vi "Calc Batch Profile Read Size.vi"(9 "Read Profile Cnt":u32, 11 "Profile Info":T1) -> (1 "Required Size(DWORD)":u32, 3 "Required Size(byte)":u32)   [LabVIEW 2010, in "KEYENCE LJ-X8000A.lvlib"]
uses:
  KEYENCE LJ-X8000A.lvlib
  Public/Clusters/Profile Info.ctl
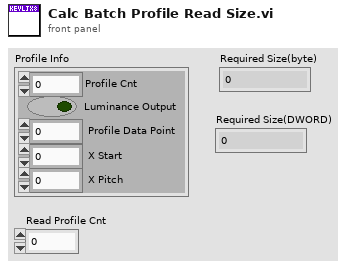
[diagram p1: front panel]
types:
  T1 = typedef "KEYENCE LJ-X8000A.lvlib/Profile Info.ctl" = cluster{"Profile Cnt":u8, "Luminance Output":bool, " Profile Data Point":u16, " X Start":i32, " X Pitch":i32}
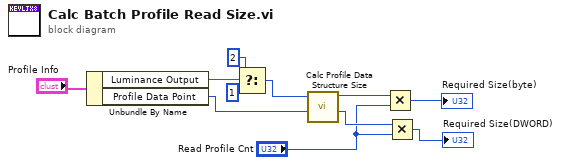
[diagram p0: block diagram]
diagram:
  n1 = Unbundle By Name("Profile Info") -> ("Luminance Output"=w6:bool, "Profile Data Point"=w10:u16)
  n2 = Select(t=u8 2 ("Profile Cnt"), s=w6, f=u8 1 ("Profile Cnt")) -> (s? t:f=w9:u8)
  n3 = call "Calc Profile Data Structure Size.vi"("Profile Data Point"=w10, "Profile Cnt"=w9) -> ("Profile Size(DWORD)"=w3:u32, "Profile Size(Byte)"=w11:u32)  [unwired: 8 in]
  n4 = Multiply(x=w11, y="Read Profile Cnt") -> (x*y=→"Required Size(byte)":u32)
  n5 = Multiply(x=w3, y="Read Profile Cnt") -> (x*y=→"Required Size(DWORD)":u32)
